vi "I32Notifier Init.vi"(8 "error in (no error)":errorcluster) -> (0 "error out":errorcluster, 3 "I32Notifier out":refnum<class "I32Notifier.lvclass">)   [LabVIEW 2018, in "I32Notifier.lvclass"]
uses:
  I32Notifier.lvclass
  I32Notifier.lvclass/I32Notifier.ctl
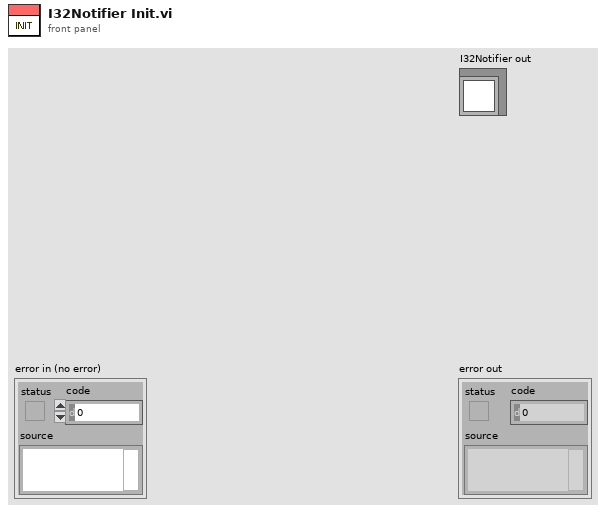
[diagram p1: front panel]
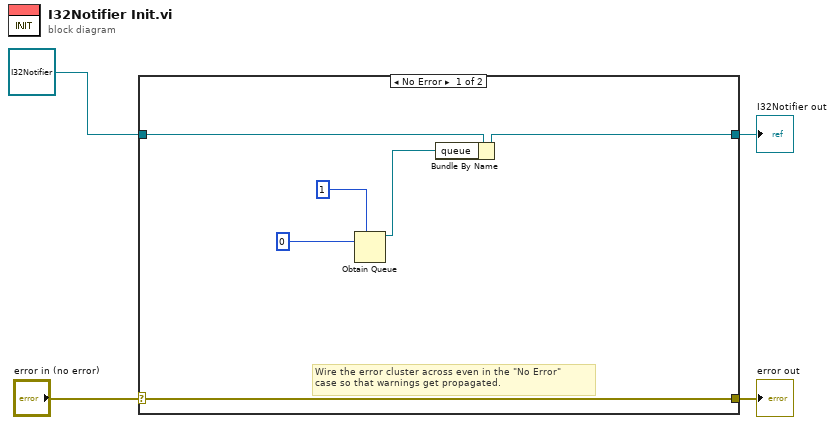
[diagram p0: block diagram]
diagram:
  n1 = case shown="No Error" "error in (no error)" {
    selector: "error in (no error)" -> [w9 w12]
    tunnel: [w9 w12] -> w3
    tunnel: [w6 w11] -> w1
    tunnel: refnum<class "I32Notifier.lvclass"> refnum ("I32Notifier in") -> [w10 w11]
    frame No Error {
      # "Wire the error cluster across even in the \"No Error\"\ncase so that warnings get propagated."
      n2 = Obtain Queue(max queue size (-1, unlimited)=1, element data type=0) -> (queue out=w5:refnum<queue>)  [unwired: 3 in, 2 out]
      n3 = Bundle By Name(cluster=w10, "queue"=w5) -> (w6:refnum<class "I32Notifier.lvclass">)
    }
    frame Error {
    }
  }
  "error out" <- w3
  "I32Notifier out" <- w1
